vi "epoll_create.vi"(8 "error in":errorcluster, 11 "epoll in":refnum<class "epoll.lvclass">) -> (0 "error out":errorcluster, 3 "epoll out":refnum<class "epoll.lvclass">)   [LabVIEW 2020, in "PCANBasic.lvlib" / "epoll.lvclass"]
doc: "This file includes code from the LinuxRT-IPC project (Apache License 2.0) https://github.com/NISystemsEngineering/LinuxRT-IPC\n\nepoll_create() creates an epoll(7) instance. Since Linux 2.6.8, the size argument is ignored, but must be greater than zero; see NOTES below.\nepoll_create() returns a file descriptor referring to the new epoll instance. This file descriptor is used for all the subsequent calls to the epoll interface. When no longer required, the file descriptor returned by epoll_create() should be closed by using close(2). When all file descriptors referring to an epoll instance have been closed, the kernel destroys the instance and releases the associated resources for reuse.\n\nepoll_create1()\nIf flags is 0, then, other than the fact that the obsolete size argument is dropped, epoll_create1() is the same as epoll_create()."
uses:
  epoll.lvclass
  epoll.lvclass/epoll.ctl
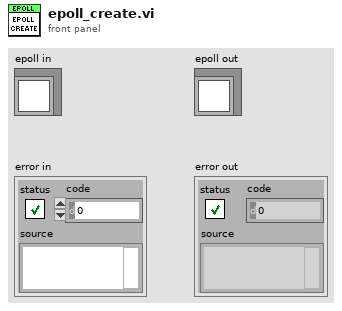
[diagram p1: front panel]
types:
  T1 = enum16{"unspecified", "close", "epoll_create", "epoll_ctl", "epoll_wait"}
  T2 = enum16{"NO ERROR", "EPERM", "ENOENT", "ESRCH", "EINTR", "EIO", "ENXIO", "E2BIG", "ENOEXEC", "EBADF", "ECHILD", "EAGAIN", "ENOMEM", "EACCES", "EFAULT", "ENOTBLK", "EBUSY", "EEXIST", "EXDEV", "ENODEV", "ENOTDIR", "EISDIR", "EINVAL", "ENFILE", "EMFILE", "ENOTTY", "ETXTBSY", "EFBIG", "ENOSPC", "ESPIPE", "EROFS", "EMLINK", "EPIPE", "EDOM", "ERANGE", "EDADLK", "ENAMETOOLONG", "ENOLCK", "ENOSYS", "ENOTEMPTY", "ELOOP", "EWOULDBLOCK", "ENOMSG", "EIDRM", "ECHRNG", "EL2NSYNC", "EL3HLT", "EL3RST", "ELNRNG", "EUNATCH", "ENOCSI", "EL2HLT", "EBADE", "EBADR", "EXFULL", "ENOANO", "EBADRQC", "EBADSLT", "EDEADLOCK", "EBFONT", "ENOSTR", "ENODATA", "ETIME", "ENOSR", "ENONET", "ENOPKG", "EREMOTE", "ENOLINK", "EADV", "ESRMNT", "ECOMM", "EPROTO", "EMULTIHOP", "EDOTDOT", "EBADMSG", "EOVERFLOW", "ENOTUNIQ", "EBADFD", "EREMCHG", "ELIBACC", "ELIBBAD", "ELIBSCN", "ELIBMAX", "ELIBEXEC", "ELISEQ", "ERESTART", "ESTRPIPE", "EUSERS", "ENOTSOCK", "EDESTADDRREQ", "EMSGSIZE", "EPROTOTYPE", "ENOPROTOOPT", "EPROTONOSUPPORT", "ESOCKTNOSUPPORT", "EOPNOTSUPP", "EPFNOSUPPORT", "EAFNOSUPPORT", "EADDRINUSE", "EADDRNOTAVAIL", "ENETDOWN", "ENETUNREACH", "ENETRESET", "ECONNABORTED", "ECONNRESET", "ENOBUFS", "EISCONN", "ENOTCONN", "ESHUTDOWN", "ETOOMANYREFS", "ETIMEDOUT", "ECONNREFUSED", "EHOSTDOWN", "EHOSTUNREACH", "EALREADY", "EINPROGRESS", "ESTALE", "EUCLEAN", "ENOTNAM", "ENAVAIL", "EISNAM", "EREMOTEIO", "EDQUOT", "ENOMEDIUM", "EMEDIUMTYPE", "ECANCELED", "ENOKEY", "EKEYEXPIRED", "EKEYREVOKED", "EKEYREJECTED", "EOWNERDEAD", "ENOTRECOVERABLE", "ERFKILL", "EHWPOISON", "UNDEFINED"}
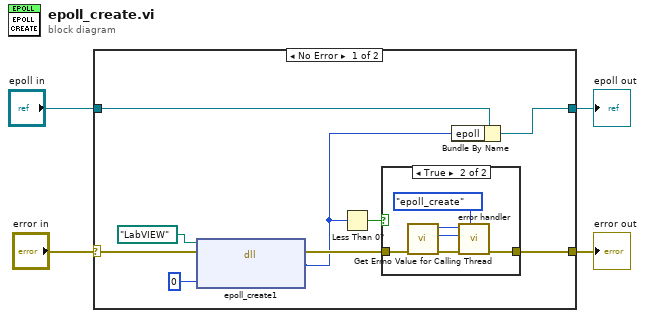
[diagram p0: block diagram]
diagram:
  n1 = case shown="No Error" "error in" {
    selector: "error in" -> [w12 w22]
    tunnel: [w8 w22] -> w3
    tunnel: [w5 w21] -> w1
    tunnel: "epoll in" -> [w9 w21]
    frame No Error {
      n2 = dll-call lib="LabVIEW" fn="epoll_create1"(path in=path "LabVIEW", error in=w12, "flags"=u16 0) -> (error out=w11:errorcluster, "fd"=w7:i32)  [unwired: 2 in, 1 out]
      n3 = Less Than 0?(x=w7) -> (x < 0?=w10:bool)
      n4 = case shown="True" w10 {
        tunnel: w11 -> [w14 w20]
        tunnel: [w14 w19] -> w8
        frame False {
        }
        frame True {
          n5 = call "Get Errno Value for Calling Thread.vi"("error in"=w20) -> ("error out"=w18:errorcluster, "errno number"=w16:i32, "errno"=w17:T2)  [unwired: 8 in]
          n6 = call "error handler.vi"("function (unspecified)"=T1."epoll_create", "error in"=w18, "errno number"=w16, "errno"=w17) -> ("error out"=w19:errorcluster)  [unwired: 7 in]
        }
      }
      n7 = Bundle By Name(cluster=w9, "epoll"=w7) -> (w5:refnum<class "epoll.lvclass">)
    }
    frame Error {
    }
  }
  "error out" <- w3
  "epoll out" <- w1
